vi "BRig_Host_comm_tcp_readAccum__v2.vi"(0 "input_handle_TCP":refnum<k5>, 2 "input_connected":bool, 5 "input_error":errorcluster, 7 "input_strAccum":string, 8 "input_I_ExpRun":bool, 9 "input_count":i32) -> (11 "output_count":i32, 13 "output_strAccum":string, 14 "output_handle_TCP":refnum<k5>, 16 "output_connected":bool, 19 "output_error":errorcluster)   [LabVIEW 2014]
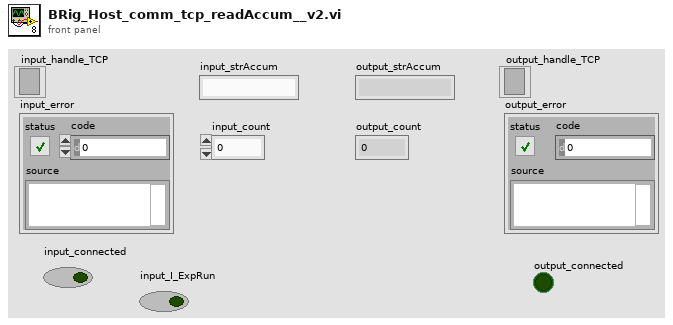
[diagram p1: front panel]
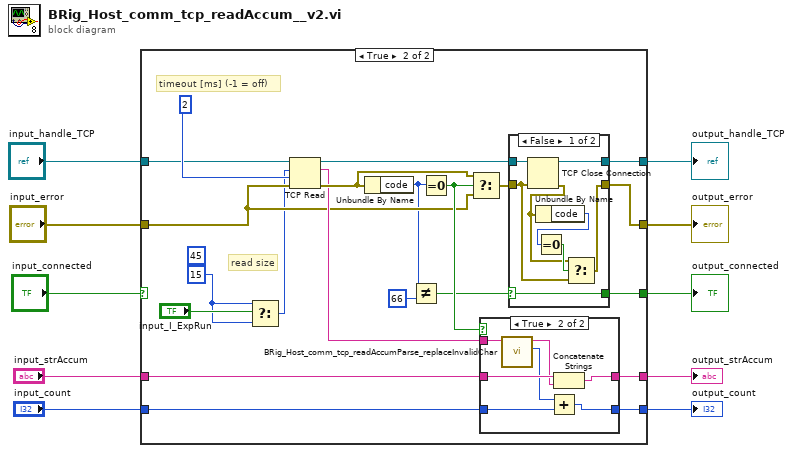
[diagram p0: block diagram]
diagram:
  n1 = case shown="True" "input_connected" {
    selector: "input_connected" -> [w11 _]
    tunnel: "input_handle_TCP" -> [w15 w35]
    tunnel: "input_error" -> [w14 w27]
    tunnel: [w14 w21] -> w8
    tunnel: "input_strAccum" -> [w13 w32]
    tunnel: [w13 w31] -> w6
    tunnel: "input_count" -> [w12 w30]
    tunnel: [w12 w29] -> w4
    tunnel: [w15 w19] -> w3
    tunnel: [w11 w23] -> w1
    frame False {
    }
    frame True {
      w16 = 15 ("bytes to read")
      (unwired) 45 ("bytes to read")
      # "read size"
      # "timeout [ms] (-1 = off)"
      n2 = Select(t=w16, s="input_I_ExpRun", f=w16) -> (s? t:f=w17:i32)
      n3 = TCP Read(connection ID=w35, bytes to read=w17, error in (no error)=w27, 9:2 ("timeout ms (25000)")) -> (connection ID out=w20:refnum<k5>, data out=w33:string, error out=w34:errorcluster)  [unwired: 1 out]
      n4 = Unbundle By Name(w34) -> ("code"=w26:i32)
      n5 = Not Equal?(x=w26, y=66) -> (x != y?=w24:bool)
      n6 = Equal To 0?(x=w26) -> (x = 0?=w28:bool)
      n7 = Select(t=w34, s=w28, f=w27) -> (s? t:f=w22:errorcluster)
      n8 = case shown="True" w28 {
        tunnel: w33 -> [_ w56]
        tunnel: w32 -> [w49 w55]
        tunnel: [w49 w51] -> w31
        tunnel: w30 -> [w48 w53]
        tunnel: [w48 w50] -> w29
        frame False {
        }
        frame True {
          n9 = call "BRig_Host_comm_tcp_readAccumParse_replaceInvalidChar.vi"("input_string"=w56) -> ("output_stringSize"=w52:i32, "output_string"=w54:string)  [unwired: 9 in]
          n10 = Add(x=w52, y=w53) -> (x+y=w50:i32)
          n11 = Concatenate Strings(w55, w54) -> (w51:string)
        }
      }
      n12 = case shown="False" w24 {
        selector: w24 -> [w42 w47]
        tunnel: [w42 w47] -> w23
        tunnel: w22 -> [w38 w46]
        tunnel: [w37 w46] -> w21
        tunnel: w20 -> [w44 w45]
        tunnel: [w43 w45] -> w19
        frame False {
          n13 = TCP Close Connection(connection ID=w44, error in (no error)=w38) -> (connection ID out=w43:refnum<k5>, error out=w39:errorcluster)  [unwired: 1 in]
          n14 = Unbundle By Name(w39) -> ("code"=w41:i32)
          n15 = Equal To 0?(x=w41) -> (x = 0?=w40:bool)
          n16 = Select(t=w39, s=w40, f=w38) -> (s? t:f=w37:errorcluster)
        }
        frame True {
        }
      }
    }
  }
  "output_handle_TCP" <- w3
  "output_error" <- w8
  "output_strAccum" <- w6
  "output_count" <- w4
  "output_connected" <- w1
